vi "RandomSequenceGenerator (SubVI).vi"(3 "Numeric":i32) -> (0 "nearest integer value":dbl, 1 "Array":dbl[](array[numeric]))   [LabVIEW 2026]
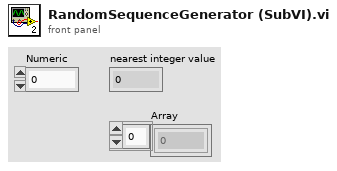
[diagram p1: front panel]
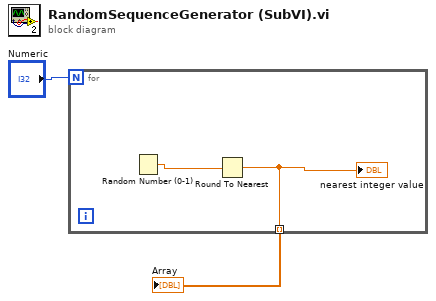
[diagram p0: block diagram]
diagram:
  n1 = for {
    N: "Numeric" -> [_]
    tunnel: [w3] -> w2 mode=indexing
    n2 = Random Number (0-1)() -> (number: 0 to 1=w4:dbl)
    n3 = Round To Nearest(number=w4) -> (nearest integer value=w3:dbl)
    "nearest integer value" <- w3
  }
  "Array" <- w2
